vi "Read Decoration.vi"(8 "error in (no error)":errorcluster, 11 "Dialog.lvclass in":refnum<class "Dialog.lvclass">) -> (0 "error out":errorcluster, 2 "Decoration":refnum<vi>, 3 "Dialog.lvclass out":refnum<class "Dialog.lvclass">)   [LabVIEW 2012, in "Dialog.lvlib" / "Dialog.lvclass"]
uses:
  Dialog.lvclass
  Dialog.lvclass/Dialog.ctl
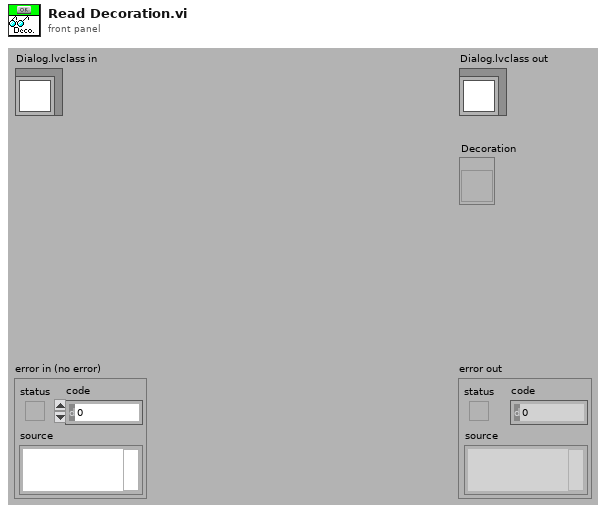
[diagram p1: front panel]
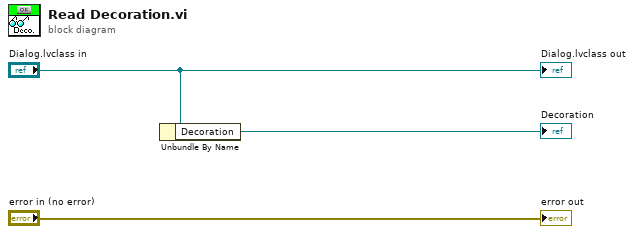
[diagram p0: block diagram]
diagram:
  n1 = Unbundle By Name("Dialog.lvclass in") -> ("Decoration"=→"Decoration":refnum<vi>)
  "error out" <- "error in (no error)"
  "Dialog.lvclass out" <- "Dialog.lvclass in"
